vi "Image Process Cal Read 2016.vi"(0 "Path":path=path "Documents/FRC/DashboardSettings.ini", 2 "PreSET Save":bool, 3 "Input cluster":T1, 4 "Save Values":bool, 5 "refnum":T2) -> (1 "file created?":bool)   [LabVIEW 2015]
uses:
  <vilib>/Utility/config.llb/Config Data RefNum.ctl
  <vilib>/Utility/config.llb/Write Key (Double).vi
  <vilib>/Utility/config.llb/Write Key (I32).vi
  <vilib>/Utility/config.llb/NI_LVConfig.lvlib
panel:
  out "error out":errorcluster
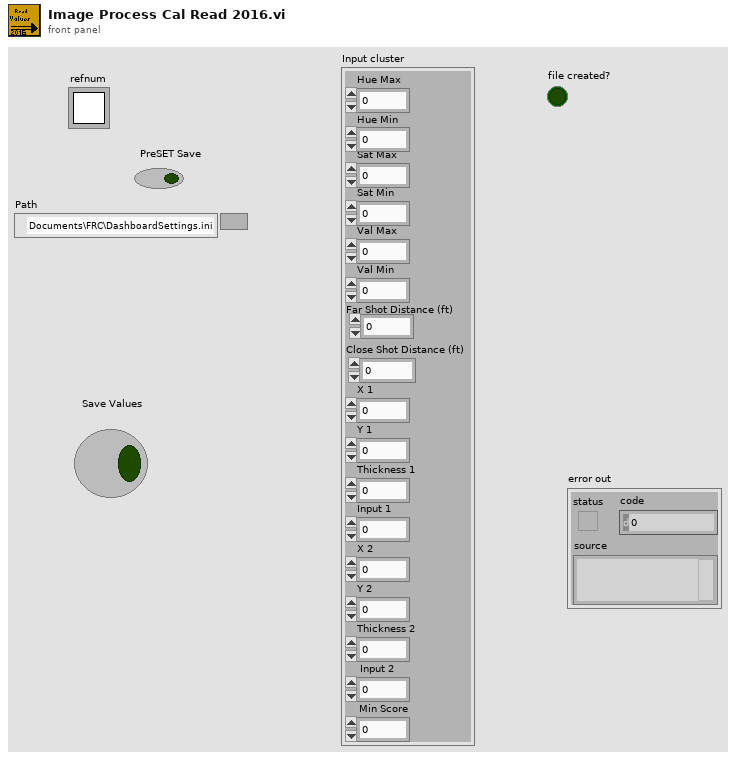
[diagram p1: front panel]
types:
  T1 = cluster{"Hue Max":dbl, "Hue Min":dbl, "Sat Max":dbl, "Sat Min":dbl, "Val Max":dbl, "Val Min":dbl, "Far Shot Distance (ft)":dbl, "Close Shot Distance (ft)":dbl, "X 1":dbl, "Y 1":i32, "Thickness 1":dbl, "Input 1":dbl, "X 2":i32, "Y 2":dbl, "Thickness 2":dbl, " Input 2    ":dbl, "Min Score":dbl}
  T2 = typedef "NI_LVConfig.lvlib/Config Data RefNum.ctl" = refnum<k1>
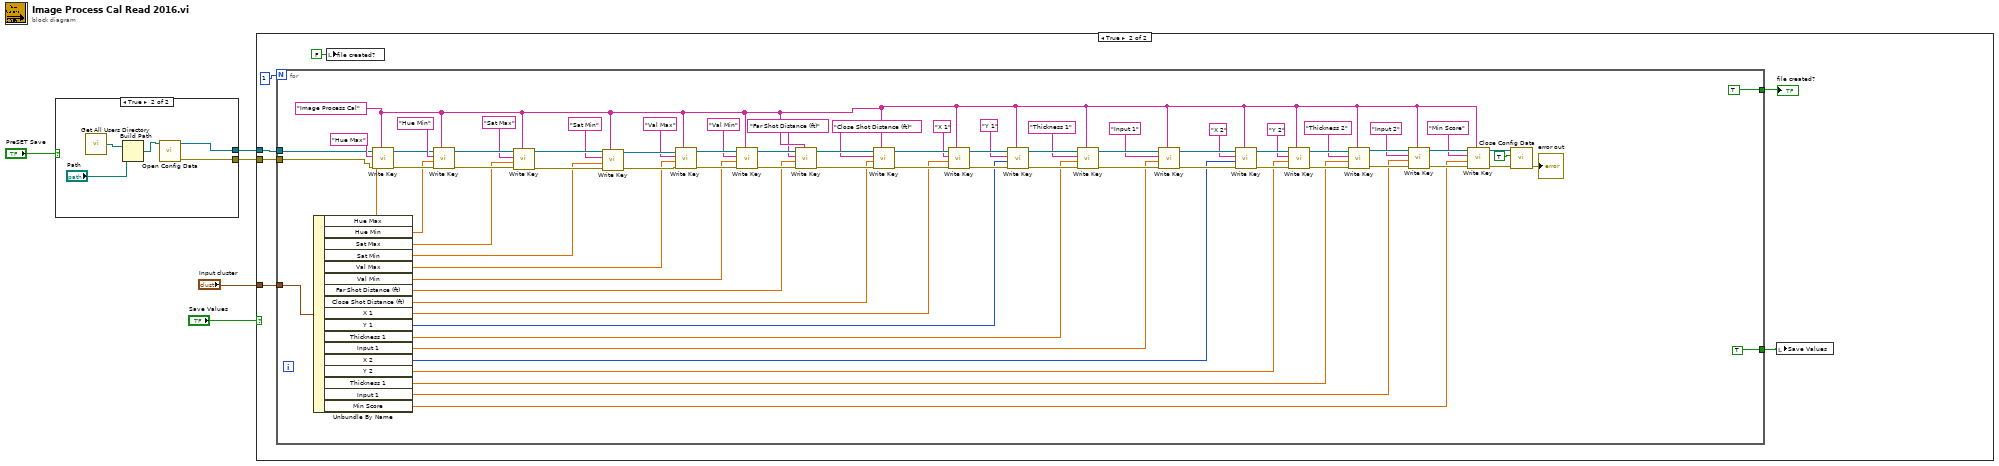
[diagram p0: block diagram]
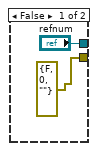
[diagram p3: hidden frame]
diagram:
  n1 = case shown="True" "PreSET Save" {
    tunnel: ["refnum" w9] -> w5
    tunnel: [errorcluster {"status"=FALSE, "code"=0, "source"=""} ("error out") w8] -> w3
    frame False {
    }
    frame True {
      n2 = call "Get All Users Directory.vi"() -> ("All User Path"=w12:path)
      n3 = Build Path(base path=w12, name or relative path="Path") -> (appended path=w10:path)
      n4 = call <vilib>:"Open Config Data.vi"("configuration file path"=w10) -> ("error out"=w8:errorcluster, "refnum"=w9:T2)  [unwired: 8 in, 1 out]
    }
  }
  n5 = case shown="True" "Save Values" {
    tunnel: w5 -> [_ w19]
    tunnel: w3 -> [_ w14]
    tunnel: "Input cluster" -> [_ w13]
    frame False {
    }
    frame True {
      n6 = for {
        N: 1 -> [_]
        tunnel: w19 -> [w80]
        tunnel: [TRUE] -> w17
        tunnel: [TRUE] -> w16
        tunnel: w14 -> [w61]
        tunnel: w13 -> [w31]
        w32 = "Image Process Cal" ("section")
        n7 = Unbundle By Name(w31) -> ("Hue Max"=w55:dbl, "Hue Min"=w54:dbl, "Sat Max"=w53:dbl, "Sat Min"=w52:dbl, "Val Max"=w51:dbl, "Val Min"=w50:dbl, "Far Shot Distance (ft)"=w49:dbl, "Close Shot Distance (ft)"=w48:dbl, "X 1"=w47:dbl, "Y 1"=w46:i32, "Thickness 1"=w45:dbl, "Input 1"=w44:dbl, "X 2"=w43:i32, "Y 2"=w36:dbl, "Thickness 1"=w35:dbl, "Input 1"=w34:dbl, "Min Score"=w33:dbl)
        n8 = call-poly <vilib>:"Write Key.vi"("section"=w32, "error in (no error)"=w61, "value"=w55, "key"="Hue Max", "refnum"=w80) -> ("error out"=w72:errorcluster, "refnum out"=w93:T2)  [unwired: 4 in, 1 out]
        n9 = call-poly <vilib>:"Write Key.vi"("section"=w32, "error in (no error)"=w72, "value"=w54, "key"="Hue Min", "refnum"=w93) -> ("error out"=w71:errorcluster, "refnum out"=w92:T2)  [unwired: 4 in, 1 out]
        n10 = call-poly <vilib>:"Write Key.vi"("section"=w32, "error in (no error)"=w71, "value"=w53, "key"="Sat Max", "refnum"=w92) -> ("error out"=w70:errorcluster, "refnum out"=w82:T2)  [unwired: 4 in, 1 out]
        n11 = call-poly <vilib>:"Write Key.vi"("section"=w32, "error in (no error)"=w70, "value"=w52, "key"="Sat Min", "refnum"=w82) -> ("error out"=w69:errorcluster, "refnum out"=w81:T2)  [unwired: 4 in, 1 out]
        n12 = call-poly <vilib>:"Write Key.vi"("section"=w32, "error in (no error)"=w69, "value"=w51, "key"="Val Max", "refnum"=w81) -> ("error out"=w68:errorcluster, "refnum out"=w90:T2)  [unwired: 4 in, 1 out]
        n13 = call-poly <vilib>:"Write Key.vi"("section"=w32, "error in (no error)"=w68, "value"=w50, "key"="Val Min", "refnum"=w90) -> ("error out"=w67:errorcluster, "refnum out"=w91:T2)  [unwired: 4 in, 1 out]
        n14 = call-poly <vilib>:"Write Key.vi"("section"=w32, "error in (no error)"=w67, "value"=w49, "key"="Far Shot Distance (ft)", "refnum"=w91) -> ("error out"=w66:errorcluster, "refnum out"=w88:T2)  [unwired: 4 in, 1 out]
        n15 = call-poly <vilib>:"Write Key.vi"("section"=w32, "error in (no error)"=w66, "value"=w48, "key"="Close Shot Distance (ft)", "refnum"=w88) -> ("error out"=w65:errorcluster, "refnum out"=w89:T2)  [unwired: 4 in, 1 out]
        n16 = call-poly <vilib>:"Write Key.vi"("section"=w32, "error in (no error)"=w65, "value"=w47, "key"="X 1", "refnum"=w89) -> ("error out"=w64:errorcluster, "refnum out"=w87:T2)  [unwired: 4 in, 1 out]
        n17 = call-poly <vilib>:"Write Key.vi"("section"=w32, "error in (no error)"=w64, "value"=w46, "key"="Y 1", "refnum"=w87) -> ("error out"=w63:errorcluster, "refnum out"=w85:T2)  [unwired: 4 in, 1 out]
        n18 = call-poly <vilib>:"Write Key.vi"("section"=w32, "error in (no error)"=w63, "value"=w45, "key"="Thickness 1", "refnum"=w85) -> ("error out"=w62:errorcluster, "refnum out"=w86:T2)  [unwired: 4 in, 1 out]
        n19 = call-poly <vilib>:"Write Key.vi"("section"=w32, "error in (no error)"=w62, "value"=w44, "key"="Input 1", "refnum"=w86) -> ("error out"=w73:errorcluster, "refnum out"=w84:T2)  [unwired: 4 in, 1 out]
        n20 = call-poly <vilib>:"Write Key.vi"("section"=w32, "error in (no error)"=w73, "value"=w43, "key"="X 2", "refnum"=w84) -> ("error out"=w56:errorcluster, "refnum out"=w57:T2)  [unwired: 4 in, 1 out]
        n21 = call-poly <vilib>:"Write Key.vi"("section"=w32, "error in (no error)"=w56, "value"=w36, "key"="Y 2", "refnum"=w57) -> ("error out"=w59:errorcluster, "refnum out"=w58:T2)  [unwired: 4 in, 1 out]
        n22 = call-poly <vilib>:"Write Key.vi"("section"=w32, "error in (no error)"=w59, "value"=w35, "key"="Thickness 2", "refnum"=w58) -> ("error out"=w39:errorcluster, "refnum out"=w40:T2)  [unwired: 4 in, 1 out]
        n23 = call-poly <vilib>:"Write Key.vi"("section"=w32, "error in (no error)"=w39, "value"=w34, "key"="Input 2", "refnum"=w40) -> ("error out"=w42:errorcluster, "refnum out"=w41:T2)  [unwired: 4 in, 1 out]
        n24 = call-poly <vilib>:"Write Key.vi"("section"=w32, "error in (no error)"=w42, "value"=w33, "key"="Min Score", "refnum"=w41) -> ("error out"=w37:errorcluster, "refnum out"=w38:T2)  [unwired: 4 in, 1 out]
        n25 = call <vilib>:"Close Config Data.vi"("error in (no error)"=w37, "write file if changed (T)"=TRUE, "refnum"=w38) -> ("error out"=→"error out":errorcluster)  [unwired: 8 out]
      }
      "file created?" <- w16
      n26 = local write "file created?"(FALSE ("file created?")) -> ()
      n27 = local write "Save Values"(w17) -> ()
    }
  }
